vi "C4If_release.vi"(0 "c4if in":refnum<k24>, 11 "error in (no error)":errorcluster) -> (15 "error out":errorcluster)   [LabVIEW 2015, in "libC4HdlLV.lvlib"]
uses:
  libC4HdlLV.lvlib
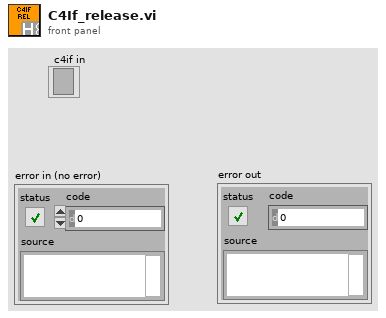
[diagram p1: front panel]
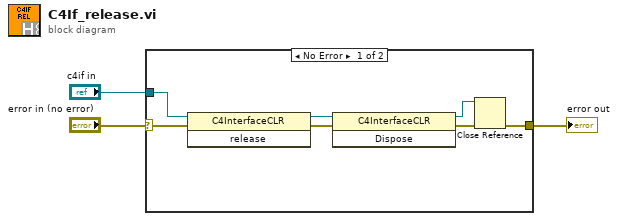
[diagram p0: block diagram]
diagram:
  n1 = case shown="No Error" "error in (no error)" {
    selector: "error in (no error)" -> [w10 w11]
    tunnel: [w5 w11] -> w3
    tunnel: "c4if in" -> [w9 _]
    frame No Error {
      n2 = invoke class="C4InterfaceCLR" method="release"(reference=w9, error in=w10) -> (reference out=w7:refnum<k24>, error out=w8:errorcluster)  [unwired: 1 in, 1 out]
      n3 = invoke class="C4InterfaceCLR" method="Dispose"(reference=w7, error in=w8) -> (reference out=w4:refnum<k24>, error out=w6:errorcluster)  [unwired: 1 in, 1 out]
      n4 = Close Reference(reference=w4, error in (no error)=w6) -> (error out=w5:errorcluster)
    }
    frame Error {
    }
  }
  "error out" <- w3
